vi "Git Commit.vi"(8 "error in (no error)":errorcluster, 10 "Commit Message":string, 11 "Git in":refnum<class "Git.lvclass">) -> (0 "error out":errorcluster, 2 "standard output":string, 3 "Git out":refnum<class "Git.lvclass">)   [LabVIEW 2019, in "Git.lvclass"]
uses:
  Git.lvclass
  Typedefs/Commands.git--combo.ctl
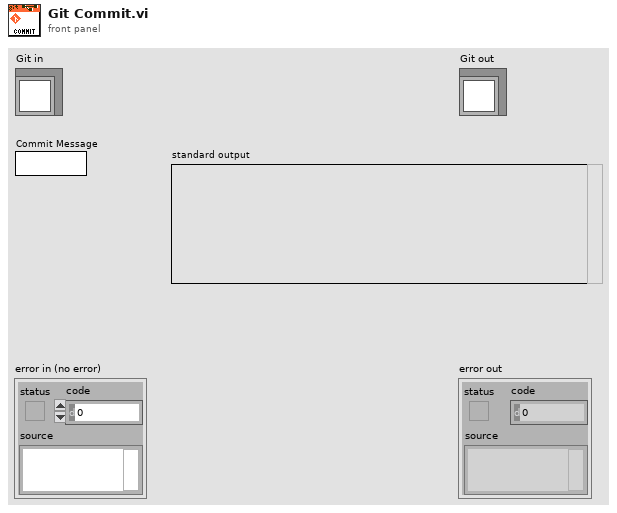
[diagram p1: front panel]
types:
  T1 = typedef "Git.lvclass/Commands.git--combo.ctl" = string
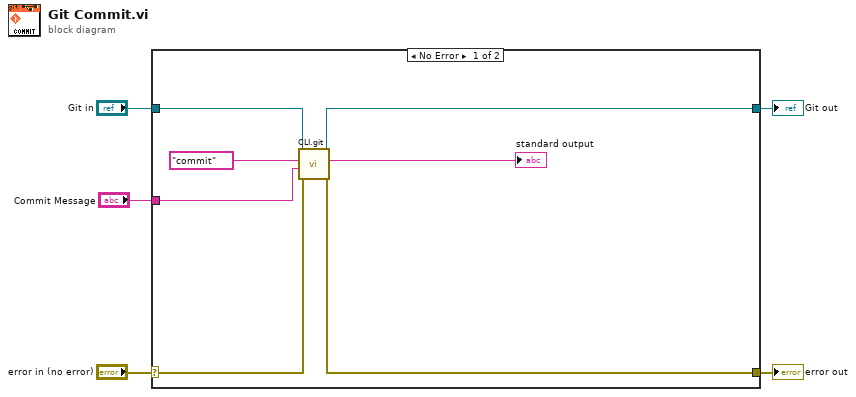
[diagram p0: block diagram]
diagram:
  n1 = case shown="No Error" "error in (no error)" {
    selector: "error in (no error)" -> [w12 w14]
    tunnel: [w11 w14] -> w4
    tunnel: [w10 w13] -> w2
    tunnel: "Git in" -> [w9 w13]
    tunnel: "Commit Message" -> [w6 _]
    frame No Error {
      n2 = call "CLI.git.vi"("error in (no error)"=w12, "Option"=w6, "Command"=T1 "commit", "Git in"=w9) -> ("error out"=w11:errorcluster, "standard output"=→"standard output":string, "Git out"=w10:refnum<class "Git.lvclass">)  [unwired: 3 in, 2 out]
    }
    frame Error {
    }
  }
  "error out" <- w4
  "Git out" <- w2
